vi "Write ExposureTime 3.vi"(8 "error in (no error)":errorcluster, 10 "ExposureTime":u32, 11 "CameraSession in":refnum<class "CS250-CameraHardwareClass.lvclass">) -> (0 "error out":errorcluster, 3 "CameraSession out":refnum<class "CS250-CameraHardwareClass.lvclass">)   [LabVIEW 2013, in "CS250-CameraHardwareClass.lvclass"]
uses:
  CS250-CameraHardwareClass.lvclass
  CS250-CameraHardwareClass.lvclass/CS250-CameraHardwareClass.ctl
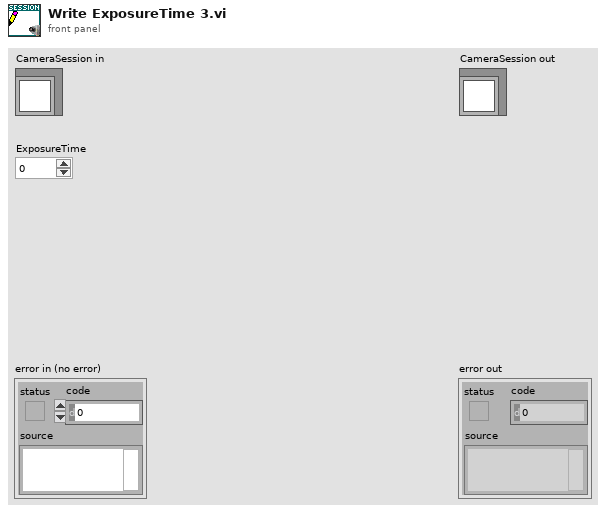
[diagram p1: front panel]
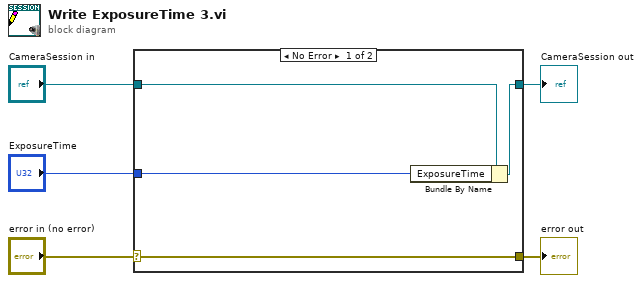
[diagram p0: block diagram]
diagram:
  n1 = case shown="No Error" "error in (no error)" {
    selector: "error in (no error)" -> [w9 w10]
    tunnel: [w9 w10] -> w4
    tunnel: [w7 w11] -> w2
    tunnel: "CameraSession in" -> [w8 w11]
    tunnel: "ExposureTime" -> [w6 _]
    frame No Error {
      n2 = Bundle By Name(cluster=w8, "ExposureTime"=w6) -> (w7:refnum<class "CS250-CameraHardwareClass.lvclass">)
    }
    frame Error {
    }
  }
  "error out" <- w4
  "CameraSession out" <- w2
